vi "Get Data.vi"(8 "error in":errorcluster, 11 "Cfg Dev in":refnum<class "Alicat Device.lvclass">) -> (0 "error out":errorcluster, 2 "DataOut":refnum<class "Data.lvclass">, 3 "Cfg Dev out":refnum<class "Alicat Device.lvclass">)   [LabVIEW 2015, in "Alicat Device.lvclass"]
uses:
  Alicat Device.lvclass
  Reusable/Data/Data.lvclass
  Alicat Device.lvclass/Alicat Device.ctl
  Data/Alicat Data.lvclass
  Reusable/Session APIs/Serial/Public/Get Data/Get String.vi
  Reusable/Session APIs/Text Communication/Text Device Session.lvclass
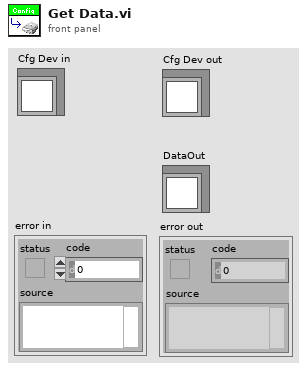
[diagram p1: front panel]
types:
  T1 = typedef "Session - Root.lvclass/Session Handle.ctl" = refnum<data-value>
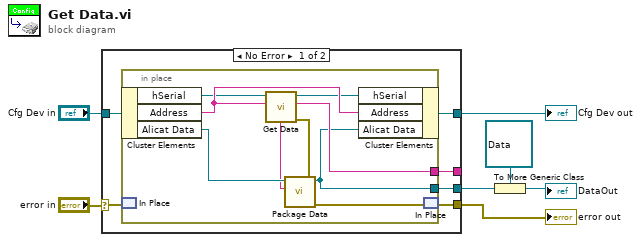
[diagram p0: block diagram]
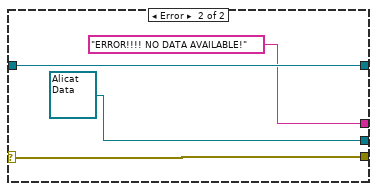
[diagram p2: hidden frame]
diagram:
  n1 = case shown="No Error" "error in" {
    selector: "error in" -> [w12 w25]
    tunnel: "Cfg Dev in" -> [w13 w24]
    tunnel: [w10 w25] -> w5
    tunnel: [w11 w24] -> w6
    tunnel: [w9 "ERROR!!!! NO DATA AVAILABLE!" ("DataOut")] -> _
    tunnel: [w8 refnum<class "Alicat Data.lvclass"> refnum ("Alicat Data out")] -> w3
    frame No Error {
      n2 = in-place {
        in-place-border: [w17] -> w9
        in-place-border: [w16] -> w8
        n3 = in-place-cluster #1(w13) -> ("hSerial"=w15:T1, "Address"=w20:string, "Alicat Data"=w21:refnum<class "Alicat Data.lvclass">)
        n4 = in-place-match #2(w12) -> ()  [unwired: 1 out]
        n5 = call-poly "Get Data.vi"("CMD"=w20, "handle in"=w15) -> ("error out"=w19:errorcluster, "DataOut"=w17:string, "handle out"=w14:T1)  [unwired: 7 in]
        n6 = call-dynamic "Package Data.vi"("error in"=w19, "DataIn"=w17, "Alicat Data in"=w21) -> ("error out"=w18:errorcluster, "Alicat Data out"=w16:refnum<class "Alicat Data.lvclass">)  [unwired: 7 in]
        n7 = in-place-cluster #1("hSerial"=w14, "Address"=w20, "Alicat Data"=w16) -> (w11:refnum<class "Alicat Device.lvclass">)
        n8 = in-place-match #2(w18) -> (w10:errorcluster)
      }
    }
    frame Error {
    }
  }
  "error out" <- w5
  "Cfg Dev out" <- w6
  n9 = To More Generic Class(target class=refnum<class "Data.lvclass"> refnum ("Base Data Lib:Data"), reference=w3) -> (generic class reference=→"DataOut":refnum<class "Data.lvclass">)
